vi "transform_translation.vi"(4 "Transform":T1) -> (1 "Translation":T1)   [LabVIEW 2013]
uses:
  <vilib>/Analysis/Matrix/Datatypes/RealMatrix.ctl
  <vilib>/Analysis/Matrix/Numeric/Conversions/Array To Matrix - RA.vi
  <vilib>/Analysis/Matrix/NI_Matrix.lvlib
panel:
  # "Extract translation part of transform matrix."
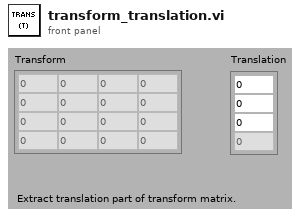
[diagram p1: front panel]
types:
  T1 = typedef "NI_Matrix.lvlib/RealMatrix.ctl" = dbl[][]
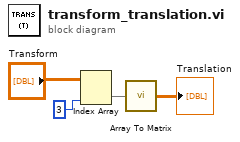
[diagram p0: block diagram]
diagram:
  n1 = Index Array(array="Transform", index (col)=3 ("disabled index (col)")) -> (element=w2:dbl[])  [unwired: 1 in]
  n2 = call-poly <vilib>:"Array To Matrix.vi"("Real 1D Array"=w2) -> ("Real Matrix (Column Vector)"=→"Translation":T1)
